vi "Enqueue Message (Single).vi"(6 "优先消息？ (F)":bool, 8 "error in (no error)":cluster{"状态":bool, "代码":i32, "源":string} caption="错误输入（无错误）", 9 "消息数据":variant, 10 "消息":string, 11 "消息队列":refnum<queue>) -> (0 "error out":cluster{"状态":bool, "代码":i32, "源":string} caption="错误输出", 3 "消息队列副本":refnum<queue>)   [LabVIEW 2018, in "Message Queue.lvlib"]
doc: "对于标准消息，将消息加入队列。对于优先消息，将消息加入队列的头部。"
uses:
  Message Queue.lvlib
  Message Cluster.ctl
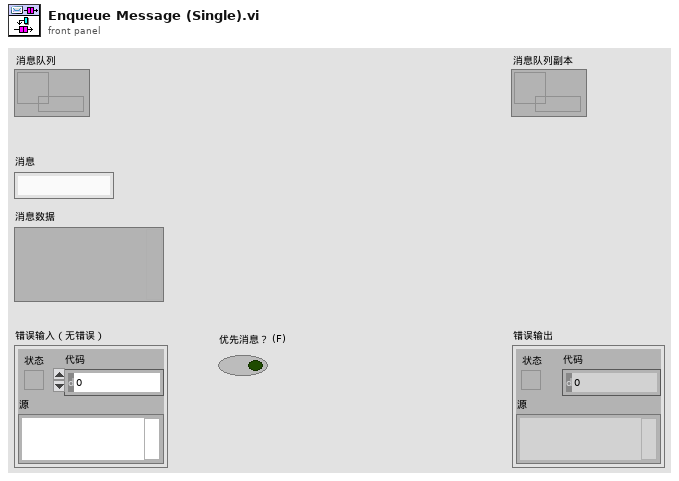
[diagram p1: front panel]
types:
  T1 = typedef "Message Queue.lvlib/Message Cluster.ctl" = cluster{"消息":string, "消息数据":variant}
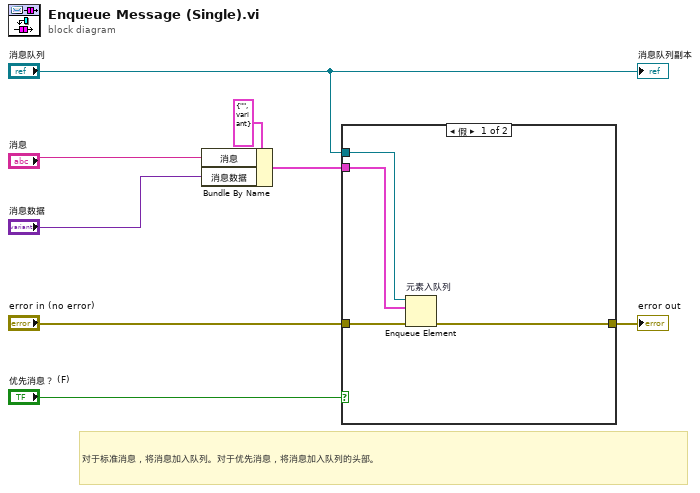
[diagram p0: block diagram]
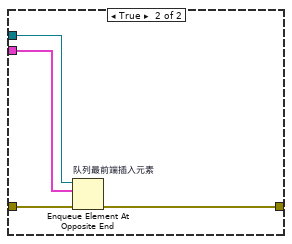
[diagram p2: hidden frame]
diagram:
  # "对于标准消息，将消息加入队列。对于优先消息，将消息加入队列的头部。"
  n1 = Bundle By Name(cluster=T1 {"消息"="", "消息数据"=variant} ("Message Cluster"), "消息"="消息", "消息数据"="消息数据") -> (w1:T1)
  n2 = case shown="假" "优先消息？ (F)" {
    tunnel: "error in (no error)" -> [w12 w16]
    tunnel: [w11 w15] -> w3
    tunnel: "消息队列" -> [w10 w14]
    tunnel: w1 -> [w9 w13]
    frame False {
      n3 = Enqueue Element "元素入队列"(queue=w10, element=w9, error in (no error)=w12) -> (error out=w11:errorcluster)  [unwired: 1 in, 2 out]
    }
    frame True {
      n4 = Enqueue Element At Opposite End "队列最前端插入元素"(queue=w14, element=w13, error in (no error)=w16) -> (error out=w15:errorcluster)  [unwired: 1 in, 2 out]
    }
  }
  "error out" <- w3
  "消息队列副本" <- "消息队列"
